vi "Exercise4.2-Pre-Lab2.vi"() -> ()   [LabVIEW 2013]
uses:
  <vilib>/Analysis/4window.llb/windowTd.ctl
  <vilib>/measure/maspectr.llb/FFT Spectrum (Mag-Phase) for 1 Chan.vi
  <vilib>/measure/NI_MABase.lvlib
  <vilib>/measure/NI_MAPro.lvlib
  <vilib>/Analysis/NI_AALPro.lvlib
panel:
  in  "Enum":T1(ring)
  out "Waveform Graph":cluster{"f0":dbl, "df":dbl, "magnitude":dbl[]}(graph)={"f0"=0.0, "df"=1.0, "magnitude"=[-346.9860547485654, -332.4102202640612, -353.84974682521397, -347.802651904699, -362.62369469253724, -358.10846228157965, -352.53817550873566, -350.20641563927677, -350.25502996485056, -345.5550362812578, -349.7419590411974, -344.6720385088076, -348.7835904979337, -344.0810228663288, -349.45356696401257, -350.69950491360487, -354.9491230807269, -370.97912368927996, -351.0611518419128, -342.826719840642, -347.1116876312752, -346.5759060349529, -356.42815622856415, -341.7170244114677, -356.99542949260535, -355.71061562949177, -348.76135223620986, -344.9337079493943, -350.4928998528824, -345.3883458659587, -350.7824574946735, -345.3764735558084, -349.970879535696, -346.17646936339884, -355.462946058808, -366.2458882894325, -355.0630925052694, -349.15886301835405, -348.4651146386312, -342.265819374179, -350.9923567234663, -342.1540971888578, -348.27233354187166, -354.572108461776, -358.52311710634217, -355.85024362323446, -351.82109820310126, -353.77804669910597, -349.80771076485655, -344.0862460080691, -347.4037401688472, -342.1640576248708, -356.0432855324972, -347.1094938727317, -354.5316100039278, -350.4436582147318, -358.483006401579, -345.0326946861974, -350.0632237709916, -340.2452383325017, -344.7803885354201, -340.9037076545238, -348.18460519127774, -359.17266524981613, -346.30640582058567, -345.6621201003529, -346.50992629644486, -342.23822318508417, -350.51311445362853, -341.99477085088915, -348.24628842003153, -338.4892736047192, -355.1363754645495, -350.92689882498985, -350.49993319417973, -345.0728249660823, -352.53852487182854, -340.75481909324856, -345.2191754330938, -347.2297239788284, -349.0731070202878, -341.4743186531933, -356.2419353694608, -357.2213248561666, -348.607453718214, -342.802656642267, -345.39240823092314, -349.18488368451904, -360.18165101264657, -347.8880769793851, -345.4371711360568, -335.46129547465216, -340.30178471272154, -341.2498950513806, -331.8593467717565, -337.17880209572536, -327.19030138294875, -339.9301142951319, -321.73016167557296, -9.03089986991943, -3.0102999566398116, -9.03089986991943, -322.3522684827159, -351.7504896989823, -327.56505385078844, -338.19835419645426, -331.40935708111266, -346.11506700517447, -339.6167509302363, -335.1419383153101, -350.26162632365157, -344.0830836017768, -355.31533539660023, -347.4171815068371, -350.6076617301156, -339.9000480563868, -365.18609731461396, -348.28061682707835, -356.13504458830306, -342.2895678866587, -354.1698377662198, -353.3938463663349, -347.2415395812668, -340.60995794229797, -349.05996439913895, -349.04301064193083, -349.5985579024347, -351.8643045355106, -358.3391679618595, -350.729038292794, -348.99422982475244, -346.21251482962145, -358.4694978731769, -343.33540266177874, -350.9158837083834, -344.3401008522111, -346.5391858100792, -357.3541661812543, -349.4486722119138, -346.02551009707736, -350.31094444797407, -341.19057093853473, -347.8309695130242, -348.81631547969954, -360.10215411259736, -348.2529977602042, -351.67021440468403, -350.40310940167984, -354.7782170617103, -337.80452203248706, -358.11198031516335, -336.80108140042245, -352.055352154971, -350.72009586033164, -348.7351067607251, -353.1912054378367, -353.5490263452024, -358.84015287581866, -348.6289142808366, -347.1749905833076, -353.9667975178311, -346.98659255475116, -358.15435778974665, -347.59950616109234, -359.84161068135114, -367.1855540064895, -354.6886680648516, -345.50564539538635, -350.55242018906495, -343.56984253187073, -351.0822958103932, -341.84854034319363, -354.67085272109364, -358.27246689606517, -352.8188825650247, -363.6123965199363, -355.2122992333185, -349.15353972843013, -357.36271871747425, -342.9021167084726, -358.02469699179574, -343.58014742500063, -350.2429290299927, -357.4256782835222, -346.8390089551333, -347.99666776905866, -351.97265230974926, -345.1431560658049, -352.38041535378807, -358.0905125283107, -355.8884110811905, -353.1134427364148, -346.782649396178, -357.22665060430216, -349.03819649225517, -352.5340295421197, -352.44286029590717, -347.6479496142756, -354.1452470783023, -335.28229915414335, -338.86532169271567, -335.59107139322697, -362.38533511056005, -351.3654843223139, -356.2882039402057, -355.11556214664597, -344.99002606163657, -357.3205287528484, -365.9442827884465, -340.8682175535086, -348.12302535074195, -343.5240923778702, -361.39445751408226, -350.5091993825906, -350.0730483935951, -358.3496679872176, -363.4596782492216, -353.04302852574347, -348.3730998567951, -348.93029099088545, -354.8814455204946, -352.3365689574922, -363.5118689750337, -349.70395539013873, -350.4694288994591, -350.6628500456784, -344.3134042575401, -346.32335652162874, -362.32784085100343, -343.7755048930736, -354.4960833118291, -344.9829577170467, -350.8377416808997, -348.0523337603674, -353.56983391670997, -353.80473063642563, -351.4428690371926, -354.31123621117615, -351.17655353583865, -346.2103423754749, -349.03529630447645, -344.1089728513461, -351.18181741798094, -348.33919227869245, -345.1521701479027, -357.84790983351104, -347.8052212147094, -351.84973787132844, -352.57403212799807, -343.87943964057763, -354.9729907942111, -343.0911312915764, -352.4692954854635, -350.92925192352914, -353.553402665033, -349.91505711577537, -359.1196223296169, -353.2513933242882, -349.9895677279656, -346.20327161815766, -358.75380978239576, -344.6748809332084, -354.9842041153207, -360.45512373504664, -356.48493140135366, -362.0140804709842, -346.1143746299206, -345.5951224512137, -350.2716146788294, -343.39535046266076, -357.99146977986396, -341.6199232875996, -352.54094220998365, -349.23297259832293, -355.3901630203567, -353.47501561120134, -370.9915233746599, -352.5233583201309, -354.7915960783876, -340.9697845894392, -355.5572275804666, -341.5489398158313, -345.98596246275895, -349.8054405906374, -347.82062288919127, -351.33575868502163, -355.0385820470631, -350.9154307297013, -352.0904219400358, -353.1137269657035, -361.73651513558195, -348.98278400142823, -349.3742331784233, -354.4178791953883, -348.2424040151318, -347.8692219624062, -352.91779140971107, -354.24808992494536, -358.2122482085811, -335.08696129992495, -327.1817669351959, -334.84909348911543, -361.6268175365624, -348.5197159245834, -347.7680776648995, -365.19482994834004, -347.13872705011744, -350.96558765813285, -349.64264723744554, -355.6720382970269, -348.42691653077117, -345.00570487444395, -351.4751568999366, -358.24194455803564, -348.088804349363, -353.7599292753156, -352.0458664288377, -353.2212557813125, -366.6129558735204, -337.970037150215, -350.81752603581543, -340.37435621847305, -351.23848497051347, -346.80964573673344, -345.8362308150631, -356.3295197173796, -355.3567032009068, -355.68161390397216, -369.76621930778947, -341.44629161294796, -355.4627559737419, -346.3042800175569, -349.0512525134136, -355.68278559775996, -351.3900033648707, -352.915044629989, -348.32568982984895, -353.8619728627124, -351.86084913411446, -336.935110532478, -347.75984919122243, -338.4216580615643, -354.37149219610046, -360.99370037959744, -358.39346774869625, -368.7022048929541, -354.6653168153632, -357.90118796506783, -355.9252349297434, -340.3724771456267, -348.64209504734094, -339.5887138652117, -358.69969231346136, -355.87800343961925, -363.85780564087975, -357.84071830851695, -353.55589836970785, -354.74650988379665, -359.92622957150434, -346.69559987654486, -348.14239291596573, -345.1745780065663, -356.53841792023286, -358.2897498406827, -369.1060055846083, -355.2320594480334, -348.2136864666312, -379.8638634953681, -360.12494797688464, -343.5121736866565, -354.14794249280635, -344.12121614047885, -352.72884362549, -363.96622932754804, -351.03944271925656, -357.2335321737365, -353.08568375029375, -354.88548935833444, -355.39522804139864, -340.0740807730244, -348.48580323083104, -340.26987035166684, -348.4011899088901, -352.17607717712605, -352.3773772786421, -356.7086502967302, -360.7171267270372, -352.15684325812686, -364.73280543014647, -349.4443201969546, -346.7324280893757, -350.93040809725346, -346.9134146945495, -355.4724807535092, -354.4374689192656, -351.547067285714, -351.71351471128605, -365.10445027453795, -349.10499706515895, -315.0290899791072, -309.3579709623739, -315.29587467491984, -347.396582253322, -350.07517131557256, -352.8127652437376, -351.09432652076055, -350.102613836838, -346.25626611385314, -356.1355748656004, -340.09640467231077, -359.47298138792127, -343.77754910896067, -356.3036313075208, -348.86272154696053, -347.0299893459665, -352.1615560365914, -352.5647852541368, -347.6950493558518, -347.9753773314149, -340.6917054356532, -349.1232190453594, -341.4426209814063, -354.88113258378775, -355.4930136855222, -352.1088339247483, -355.4743359067357, -352.680167609886, -370.3188434082939, -357.29295162176834, -351.21647375261955, -349.6298662011118, -364.35318176199956, -348.95175715236667, -346.6903042055947, -350.7605481969602, -354.5163768915737, -355.5056397337761, -360.1936074406313, -376.1174517193487, -348.6672111653529, -358.58099061034665, -350.3564132216516, -350.28041928459777, -347.85433049415485, -350.10283774116, -356.3043973529369, -350.6208598210561, -350.87774991948083, -350.01555918176086, -355.89681166858566, -349.6836894962743, -355.16850791462923, -363.206486426316, -358.3251062471221, -347.62612906595007, -349.66888672907896, -360.008801768985, -350.1309110690087, -348.2407729689934, -340.2767066789945, -345.27056637515614, -338.8280220537845, -360.6725166720362, -363.96399535291687, -352.6442976218631, -364.8793526321634, -352.22796205363096, -352.2605047024127, -348.04533807474877, -348.41653312468276, -346.78479343623025, -342.7430050359309, -357.05384313660596, -351.7680365263141, -357.1988553594696, -362.76052055128156, -348.3970800474573, -350.61301958430926, -354.5397891228024, -336.7549320017804, -350.22812482918516, -336.8643834004985, -347.3093514722889, -345.8469426125282, -349.3573418284933, -359.0603945273425, -360.0009143728171, -370.23294387797796, -354.18179105008784, -349.91354343576063, -345.55413699612825, -346.04663775685594, -346.4404894762305, -349.6004068420388, -349.13717644530516, -354.3661829559846, -351.7588904699925, -350.11205792892656, -358.0768532836094, -342.88435437796693]}
  in  "window":T2=1 items=["Rectangle"=0, "Hanning"=1, "Hamming"=2, "Blackman-Harris"=3, "Exact Blackman"=4, "Blackman"=5, "Flat Top"=6, "4 Term B-Harris "=7, "7 Term B-Harris"=8, "Low Sidelobe"=9, "Blackman Nuttall"=11, "Triangle"=30, "Bartlett-Hanning"=31, "Bohman"=32, "Parzen"=33, "Welch"=34, "Kaiser"=60, "Dolph-Chebyshev"=61, "Gaussian"=62]
  in  "stop":bool
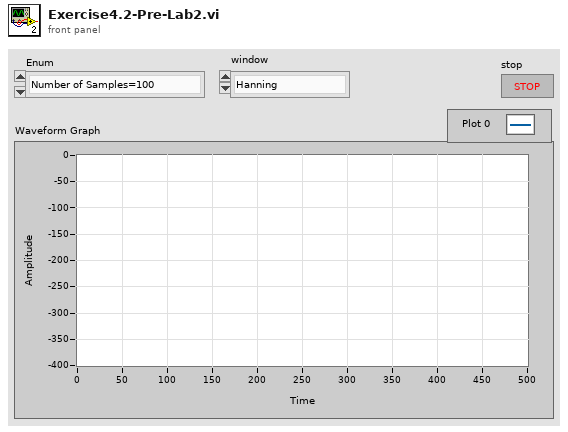
[diagram p1: front panel]
types:
  T1 = enum16{"Number of Samples=100", "Number of Samples=400", "Number of Samples=1000", "Number of Samples=996"}
  T2 = typedef "NI_AALPro.lvlib/windowTd.ctl" = u32
  T3 = cluster{"dB On (F)":bool, "unwrap phase (F)":bool, "convert to degree (F)":bool}
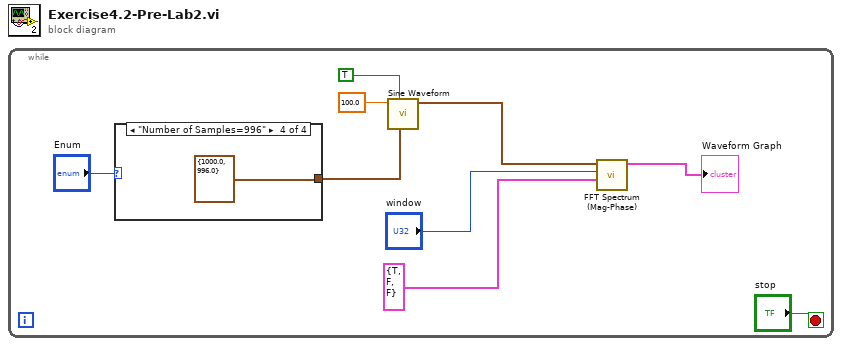
[diagram p0: block diagram]
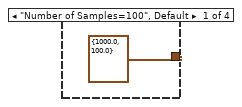
[diagram p2: hidden frame]
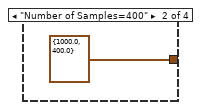
[diagram p3: hidden frame]
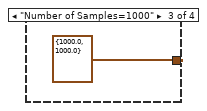
[diagram p4: hidden frame]
diagram:
  n1 = while {
    stop <- "stop" stop-if-true
    n2 = case shown="\"Number of Samples=996\"" "Enum" {
      tunnel: [cluster{"Fs":dbl, "#s":dbl} {"Fs"=1000.0, "#s"=100.0} ("sampling info") cluster{"Fs":dbl, "#s":dbl} {"Fs"=1000.0, "#s"=400.0} ("sampling info") cluster{"Fs":dbl, "#s":dbl} {"Fs"=1000.0, "#s"=1000.0} ("sampling info") cluster{"Fs":dbl, "#s":dbl} {"Fs"=1000.0, "#s"=996.0} ("sampling info")] -> w2
      frame "Number of Samples=100", Default {
      }
      frame "Number of Samples=400" {
      }
      frame "Number of Samples=1000" {
      }
      frame "Number of Samples=996" {
      }
    }
    n3 = call <vilib>:"Sine Waveform.vi"("sampling info"=w2, "reset signal"=TRUE, "frequency"=100.0) -> ("signal out"=w8:waveform(dbl))  [unwired: 7 in, 1 out]
    n4 = call-poly <vilib>:"FFT Spectrum (Mag-Phase).vi"("view"=T3 {"dB On (F)"=TRUE, "unwrap phase (F)"=FALSE, "convert to degree (F)"=FALSE}, "window"="window", "time signal"=w8) -> ("magnitude"=→"Waveform Graph":cluster{"f0":dbl, "df":dbl, "magnitude":dbl[]})  [unwired: 4 in, 4 out]
  }
